vi "DC_Link_v1.vi"(8 "error in":errorcluster) -> (0 "error out":errorcluster, 3 "DC Gain":dbl[](array[numeric]))   [LabVIEW 2022 SP3]
uses:
  <vilib>/DAQmx/write.llb/DAQmx Write (Analog 1D Wfm NChan NSamp).vi
  <vilib>/DAQmx/read.llb/DAQmx Read (Analog 1D Wfm NChan NSamp).vi
  <vilib>/DAQmx/write.llb/DAQmx Write (Analog 1D DBL NChan 1Samp).vi
  <vilib>/DAQmx/create/channels.llb/DAQmx Create Channel (AO-Voltage-Basic).vi
  <vilib>/DAQmx/configure/timing.llb/DAQmx Timing (Sample Clock).vi
  <vilib>/measure/madcrms.llb/Basic Averaged DC-RMS for N Chan.vi
  <vilib>/DAQmx/miscellaneous.llb/DAQmx Fill In Error Info.vi
  <resource>/objmgr/daqmx.rc
  <vilib>/measure/NI_MABase.lvlib
  <vilib>/measure/NI_MAPro.lvlib
panel:
  out "Output Signal":waveform(dbl)[](graph)
  out "Input Signal":waveform(dbl)[](graph)
  in  "Number of Samples 2":i32=1000
  in  "Sample Rate 2":dbl=1000.0
  in  "Signal 1 (5V)":tag="OnboardClock"
  out "Actual Sample Rate 2":dbl=1000.0 format="%0.2f"
  # "This test will input inverse waveforms into the DC Link -/+"
  # "And capture the DC Link Voltage, as well as the Overvoltage Fault"
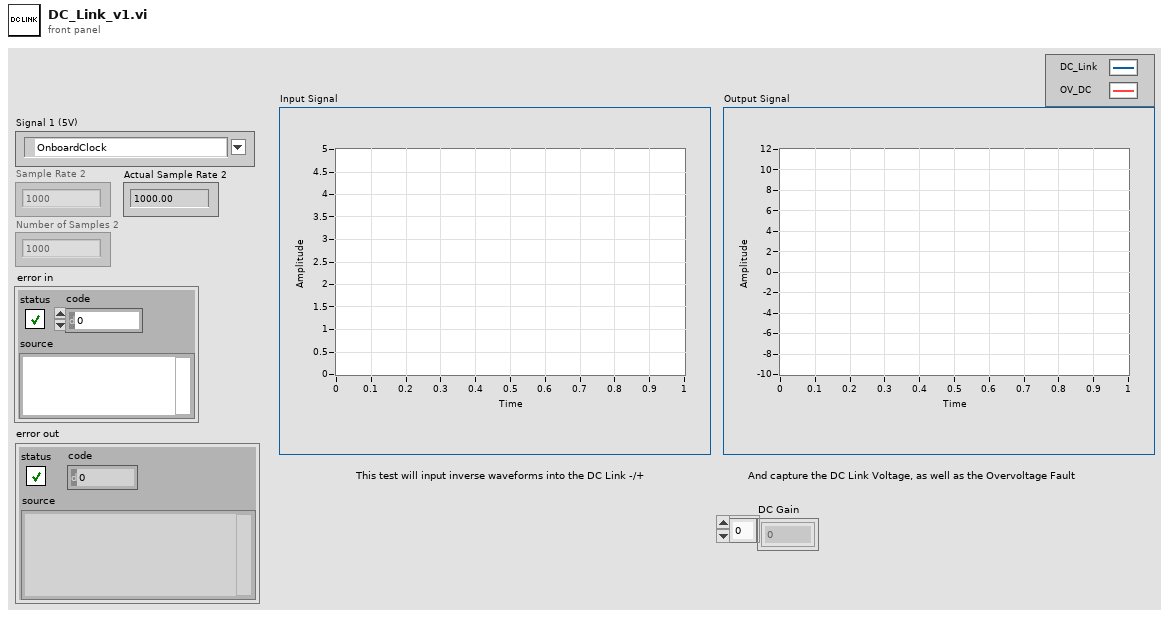
[diagram p1: front panel]
types:
  T1 = cluster{"Waveform Type":u16, "Amplitude":dbl, "Frequency":dbl}[]
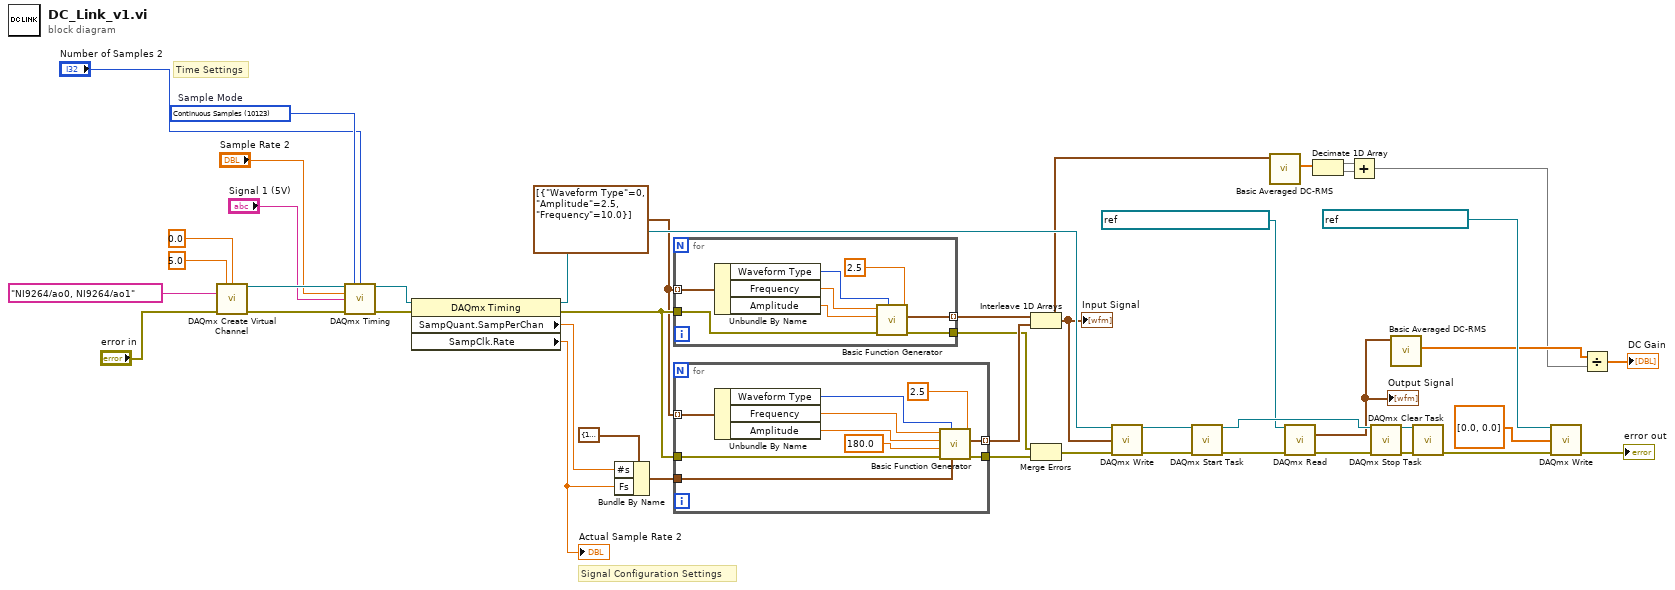
[diagram p0: block diagram]
diagram:
  w14 = T1 [{"Waveform Type"=0, "Amplitude"=2.5, "Frequency"=10.0}] ("Signal Input")
  w34 = 10123 items=["Finite Samples"=10178, "Continuous Samples"=10123, "Hardware Timed Single Point"=12522]  # Sample Mode
  # "Time Settings"
  # "Signal Configuration Settings"
  n1 = call-poly <vilib>:"DAQmx Create Virtual Channel.vi"("maximum value"=5.0, "minimum value"=0.0, "physical channels"=tag "NI9264/ao0, NI9264/ao1", "error in"="error in") -> ("task out"=w32:refnum<k21>, "error out"=w33:errorcluster)  [unwired: 10 in]
  n2 = call-poly <vilib>:"DAQmx Timing.vi"("task/channels in"=w32, "sample mode"=w34, "samples per channel"="Number of Samples 2", "rate"="Sample Rate 2", "source"="Signal 1 (5V)", "error in"=w33) -> ("task out"=w36:refnum<k21>, "error out"=w35:errorcluster)  [unwired: 8 in]
  n3 = property class="DAQmx Timing"(reference=w36, error in=w35) -> (reference out=w44:refnum<k21>, error out=w21:errorcluster, "SampQuant.SampPerChan"=w27:dbl, "SampClk.Rate"=w26:dbl)
  "Actual Sample Rate 2" <- w26
  n4 = Bundle By Name(cluster=cluster{"Fs":dbl, "#s":dbl} {"Fs"=1000.0, "#s"=1000.0} ("sampling info"), "#s"=w27, "Fs"=w26) -> (w22:cluster{"Fs":dbl, "#s":dbl})
  n5 = for {
    tunnel: [w52] -> w17
    tunnel: w14 -> [w51] mode=indexing
    tunnel: [w47] -> w37 mode=indexing
    tunnel: w21 -> [w46]
    n6 = Unbundle By Name(w51) -> ("Waveform Type"=w50:u16, "Frequency"=w49:dbl, "Amplitude"=w48:dbl)
    n7 = call <vilib>:"Basic Function Generator.vi"("offset"=2.5, "signal type"=w50, "error in (no error)"=w46, "amplitude"=w48, "frequency"=w49) -> ("error out"=w52:errorcluster, "signal out"=w47:waveform(dbl))  [unwired: 4 in, 1 out]
  }
  n8 = for {
    tunnel: w21 -> [w55]
    tunnel: w22 -> [w62]
    tunnel: [w61] -> w16
    tunnel: w14 -> [w60] mode=indexing
    tunnel: [w56] -> w43 mode=indexing
    n9 = Unbundle By Name(w60) -> ("Waveform Type"=w59:u16, "Frequency"=w58:dbl, "Amplitude"=w57:dbl)
    n10 = call <vilib>:"Basic Function Generator.vi"("offset"=2.5, "sampling info"=w62, "signal type"=w59, "error in (no error)"=w55, "phase"=180.0, "amplitude"=w57, "frequency"=w58) -> ("error out"=w61:errorcluster, "signal out"=w56:waveform(dbl))  [unwired: 2 in, 1 out]
  }
  n11 = Interleave 1D Arrays(w37, w43) -> (w8:waveform(dbl)[])
  "Input Signal" <- w8
  n12 = Merge Errors(w17, w16) -> (w15:errorcluster)
  n13 = call-poly <vilib>:"DAQmx Write.vi"("task/channels in"=w44, "data"=w8, "error in"=w15) -> ("task out"=w42:refnum<k21>, "error out"=w41:errorcluster)  [unwired: 10 in, 1 out]
  n14 = call <vilib>:"DAQmx Start Task.vi"("task/channels in"=w42, "error in"=w41) -> ("task out"=w39:refnum<k21>, "error out"=w40:errorcluster)  [unwired: 12 in]
  n15 = call-poly <vilib>:"Basic Averaged DC-RMS.vi"("signals in"=w8) -> ("RMS values"=w6:dbl[])  [unwired: 7 in, 3 out]
  n16 = call-poly <vilib>:"DAQmx Read.vi"("task/channels in"=refnum<k21> "BONTS_DC-Link_Feedback", "error in"=w40) -> ("data"=w7:waveform(dbl)[], "error out"=w38:errorcluster)  [unwired: 11 in, 1 out]
  "Output Signal" <- w7
  n17 = Decimate 1D Array(w6) -> (w5:dbl[], w4:dbl[])
  n18 = Add(x=w5, y=w4) -> (x+y=w2:dbl[])
  n19 = call <vilib>:"DAQmx Stop Task.vi"("task/channels in"=w39, "error in"=w38) -> ("task out"=w18:refnum<k21>, "error out"=w19:errorcluster)  [unwired: 12 in]
  n20 = call-poly <vilib>:"Basic Averaged DC-RMS.vi"("signals in"=w7) -> ("RMS values"=w3:dbl[])  [unwired: 7 in, 3 out]
  n21 = call <vilib>:"DAQmx Clear Task.vi"("task in"=w18, "error in"=w19) -> ("error out"=w10:errorcluster)  [unwired: 13 in]
  n22 = call-poly <vilib>:"DAQmx Write.vi"("task/channels in"=refnum<k21> "BONTS_DC-Link_Input", "data"=dbl[] [0.0, 0.0], "error in"=w10) -> ("error out"=→"error out":errorcluster)  [unwired: 10 in, 2 out]
  n23 = Divide(x=w3, y=w2) -> (x/y=→"DC Gain":dbl[])
